vi "Lab Panel V4.91.vi"() -> ()   [LabVIEW 2013] (continued)
                n1771 = property on="SET LAB03-2" class="Clust (strict)"("DisabledEnum"=w3330) -> ()  [unwired: 2 in, 2 out]
                n1772 = property on="SET LAB04-1" class="Clust (strict)"("DisabledEnum"=w3329) -> ()  [unwired: 2 in, 2 out]
                n1773 = property on="SET LAB04-2" class="Clust (strict)"("DisabledEnum"=w3328) -> ()  [unwired: 2 in, 2 out]
                n1774 = property on="O/I  LAB05-2" class="Bool (strict)"("DisabledEnum"=w3326) -> ()  [unwired: 2 in, 2 out]
                n1775 = property on="O/I  LAB05-1" class="Bool (strict)"("DisabledEnum"=w3327) -> ()  [unwired: 2 in, 2 out]
                n1776 = property on="O/I  LAB04-1" class="Bool (strict)"("DisabledEnum"=w3329) -> ()  [unwired: 2 in, 2 out]
                n1777 = property on="O/I  LAB04-2" class="Bool (strict)"("DisabledEnum"=w3328) -> ()  [unwired: 2 in, 2 out]
                n1778 = property on="O/I  LAB03-2" class="Bool (strict)"("DisabledEnum"=w3330) -> ()  [unwired: 2 in, 2 out]
                n1779 = Not(x=w3335) -> (.not. x?=w3336:bool)
                n1780 = Not(x=w3334) -> (.not. x?=w3337:bool)
                n1781 = Not(x=w3333) -> (.not. x?=w3338:bool)
                n1782 = property on="RESULT LAB05-2" class="Bool (strict)"("Visible"=w3336) -> ()  [unwired: 2 in, 2 out]
                n1783 = property on="RESULT LAB05-1" class="Bool (strict)"("Visible"=w3337) -> ()  [unwired: 2 in, 2 out]
                n1784 = Not(x=w3332) -> (.not. x?=w3339:bool)
                n1785 = property on="RESULT LAB04-2" class="Bool (strict)"("Visible"=w3338) -> ()  [unwired: 2 in, 2 out]
                n1786 = Not(x=w3331) -> (.not. x?=w3340:bool)
                n1787 = property on="RESULT LAB04-1" class="Bool (strict)"("Visible"=w3339) -> ()  [unwired: 2 in, 2 out]
                n1788 = property on="RESULT LAB03-2" class="Bool (strict)"("Visible"=w3340) -> ()  [unwired: 2 in, 2 out]
              }
              frame #2 {
                # "disable calibrate if any test running"
                n1789 = Or(x=w3363, y=w3362) -> (x .or. y?=w3356:bool)
                n1790 = Or(x=w3365, y=w3364) -> (x .or. y?=w3358:bool)
                n1791 = Or(x=w3369, y=w3368) -> (x .or. y?=w3360:bool)
                n1792 = Or(x=w3367, y=w3366) -> (x .or. y?=w3359:bool)
                n1793 = Or(x=w3371, y=w3370) -> (x .or. y?=w3361:bool)
                n1794 = Or(x=w3359, y=w3358) -> (x .or. y?=w3357:bool)
                n1795 = Or(x=w3361, y=w3360) -> (x .or. y?=w3355:bool)
                n1796 = Or(x=w3357, y=w3356) -> (x .or. y?=w3354:bool)
                n1797 = Or(x=w3355, y=w3354) -> (x .or. y?=w3353:bool)
                n1798 = case shown="False" w3353 {
                  tunnel: [0 2] -> w3352
                  frame False {
                  }
                  frame True {
                  }
                }
                n1799 = property on="JIG TEST" class="Clust (strict)"("DisabledEnum"=w3352) -> ()  [unwired: 2 in, 2 out]
                n1800 = property on="Network Directory" class="Path"("DisabledEnum"=w3352) -> ()  [unwired: 2 in, 2 out]
                n1801 = property on="MAIL SETTINGS" class="Clust (strict)"("DisabledEnum"=w3352) -> ()  [unwired: 2 in, 2 out]
                n1802 = property on="SET (cal)" class="Bool (strict)"("DisabledEnum"=w3352) -> ()  [unwired: 2 in, 2 out]
                n1803 = property on="ADMIN" class="Bool (strict)"("DisabledEnum"=0) -> ()  [unwired: 2 in, 2 out]
              }
            }
          }
          frame #8 {
            # "drive jigs"
            n1804 = stacked-sequence {
              frame #0 {
                # "jig on"
                n1805 = local read "jig cycle"() -> (w3379:dbl)
                n1806 = property on="JIG TEST" class="Clust (strict)"() -> ("DisabledEnum"=w3376:T16)  [unwired: 2 in, 2 out]
                n1807 = Equal?(x=w3376, y=2) -> (x = y?=w3375:bool)
                n1808 = Equal?(x=w3379, y=0) -> (x = y?=w3377:bool)
                n1809 = And(x=w3377, y=w3375) -> (x .and. y?=w3374:bool)
                n1810 = case shown="True" w3374 {
                  frame False {
                  }
                  frame True {
                    n1811 = local read "run lab01-1"() -> (w3390:bool)
                    n1812 = local read "run lab01-2"() -> (w3389:bool)
                    n1813 = local read "run lab02-1"() -> (w3388:bool)
                    n1814 = local read "run lab02-2"() -> (w3387:bool)
                    n1815 = local read "run lab03-1"() -> (w3386:bool)
                    n1816 = local read "run lab03-2"() -> (w3385:bool)
                    n1817 = local read "run lab04-1"() -> (w3384:bool)
                    n1818 = local read "run lab04-2"() -> (w3383:bool)
                    n1819 = local read "run lab05-1"() -> (w3382:bool)
                    n1820 = local read "run lab05-2"() -> (w3381:bool)
                    n1821 = local write "JIG LAB03-2"(w3385) -> ()
                    n1822 = local write "JIG LAB01-1"(w3390) -> ()
                    n1823 = local write "JIG LAB01-2"(w3389) -> ()
                    n1824 = local write "JIG LAB02-1"(w3388) -> ()
                    n1825 = local write "JIG LAB02-2"(w3387) -> ()
                    n1826 = local write "JIG LAB03-1"(w3386) -> ()
                    n1827 = local write "JIG LAB04-1"(w3384) -> ()
                    n1828 = local write "JIG LAB04-2"(w3383) -> ()
                    n1829 = local write "JIG LAB05-1"(w3382) -> ()
                    n1830 = local write "JIG LAB05-2"(w3381) -> ()
                  }
                }
              }
              frame #1 {
                # "jig off"
                n1831 = local read "jig cycle"() -> (w3397:dbl)
                n1832 = local read "on loops"() -> (w3396:dbl)
                n1833 = property on="JIG TEST" class="Clust (strict)"() -> ("DisabledEnum"=w3395:T16)  [unwired: 2 in, 2 out]
                n1834 = Equal?(x=w3395, y=2) -> (x = y?=w3393:bool)
                n1835 = Equal?(x=w3397, y=w3396) -> (x = y?=w3392:bool)
                n1836 = And(x=w3392, y=w3393) -> (x .and. y?=w3391:bool)
                n1837 = case shown="True" w3391 {
                  frame False {
                  }
                  frame True {
                    w3448 = FALSE
                    w3449 = TRUE
                    w3447 = 2
                    n1838 = local read "SELECT LAB05-2"() -> (w3438:T3)
                    n1839 = local read "SELECT LAB04-2"() -> (w3440:T3)
                    n1840 = local read "SELECT LAB04-1"() -> (w3441:T3)
                    n1841 = local read "SELECT LAB05-1"() -> (w3439:T3)
                    n1842 = local read "SELECT LAB03-2"() -> (w3442:T3)
                    n1843 = local read "SELECT LAB02-1"() -> (w3445:T3)
                    n1844 = local read "SELECT LAB03-1"() -> (w3443:T3)
                    n1845 = local read "SELECT LAB02-2"() -> (w3444:T3)
                    n1846 = local read "SELECT LAB01-2"() -> (w3446:T3)
                    n1847 = local read "run lab05-1"() -> (w3408:bool)
                    n1848 = local read "run lab05-2"() -> (w3407:bool)
                    n1849 = local read "SELECT LAB01-1"() -> (w3450:T3)
                    n1850 = local read "run lab04-2"() -> (w3409:bool)
                    n1851 = local read "run lab04-1"() -> (w3410:bool)
                    n1852 = local read "run lab01-1"() -> (w3426:bool)
                    n1853 = local read "run lab01-2"() -> (w3415:bool)
                    n1854 = local read "run lab03-2"() -> (w3411:bool)
                    n1855 = local read "run lab03-1"() -> (w3412:bool)
                    n1856 = local read "run lab02-1"() -> (w3414:bool)
                    n1857 = local read "run lab02-2"() -> (w3413:bool)
                    n1858 = Equal?(x=w3447, y=w3443) -> (x = y?=w3421:bool)
                    n1859 = Equal?(x=w3447, y=w3442) -> (x = y?=w3420:bool)
                    n1860 = Equal?(x=w3447, y=w3441) -> (x = y?=w3419:bool)
                    n1861 = Equal?(x=w3447, y=w3440) -> (x = y?=w3418:bool)
                    n1862 = Equal?(x=w3447, y=w3439) -> (x = y?=w3417:bool)
                    n1863 = Equal?(x=w3447, y=w3438) -> (x = y?=w3416:bool)
                    n1864 = Equal?(x=w3447, y=w3450) -> (x = y?=w3427:bool)
                    n1865 = Equal?(x=w3447, y=w3445) -> (x = y?=w3423:bool)
                    n1866 = Equal?(x=w3447, y=w3444) -> (x = y?=w3422:bool)
                    n1867 = Equal?(x=w3447, y=w3446) -> (x = y?=w3424:bool)
                    n1868 = And(x=w3418, y=w3409) -> (x .and. y?=w3400:bool)
                    n1869 = And(x=w3421, y=w3412) -> (x .and. y?=w3403:bool)
                    n1870 = And(x=w3419, y=w3410) -> (x .and. y?=w3401:bool)
                    n1871 = And(x=w3416, y=w3407) -> (x .and. y?=w3398:bool)
                    n1872 = And(x=w3422, y=w3413) -> (x .and. y?=w3404:bool)
                    n1873 = And(x=w3420, y=w3411) -> (x .and. y?=w3402:bool)
                    n1874 = And(x=w3417, y=w3408) -> (x .and. y?=w3399:bool)
                    n1875 = And(x=w3424, y=w3415) -> (x .and. y?=w3406:bool)
                    n1876 = And(x=w3427, y=w3426) -> (x .and. y?=w3425:bool)
                    n1877 = And(x=w3423, y=w3414) -> (x .and. y?=w3405:bool)
                    n1878 = Select(t=w3449, s=w3425, f=w3448) -> (s? t:f=w3428:bool)
                    n1879 = Select(t=w3449, s=w3406, f=w3448) -> (s? t:f=w3429:bool)
                    n1880 = Select(t=w3449, s=w3405, f=w3448) -> (s? t:f=w3430:bool)
                    n1881 = Select(t=w3449, s=w3404, f=w3448) -> (s? t:f=w3431:bool)
                    n1882 = Select(t=w3449, s=w3403, f=w3448) -> (s? t:f=w3432:bool)
                    n1883 = Select(t=w3449, s=w3402, f=w3448) -> (s? t:f=w3433:bool)
                    n1884 = Select(t=w3449, s=w3401, f=w3448) -> (s? t:f=w3434:bool)
                    n1885 = Select(t=w3449, s=w3400, f=w3448) -> (s? t:f=w3435:bool)
                    n1886 = Select(t=w3449, s=w3399, f=w3448) -> (s? t:f=w3436:bool)
                    n1887 = Select(t=w3449, s=w3398, f=w3448) -> (s? t:f=w3437:bool)
                    n1888 = local write "JIG LAB03-2"(w3433) -> ()
                    n1889 = local write "JIG LAB02-1"(w3430) -> ()
                    n1890 = local write "JIG LAB02-2"(w3431) -> ()
                    n1891 = local write "JIG LAB01-2"(w3429) -> ()
                    n1892 = local write "JIG LAB03-1"(w3432) -> ()
                    n1893 = local write "JIG LAB01-1"(w3428) -> ()
                    n1894 = local write "JIG LAB05-2"(w3437) -> ()
                    n1895 = local write "JIG LAB04-1"(w3434) -> ()
                    n1896 = local write "JIG LAB05-1"(w3436) -> ()
                    n1897 = local write "JIG LAB04-2"(w3435) -> ()
                  }
                }
              }
            }
          }
          frame #9 {
            # "enable  jig test output if no test busy"
            n1898 = property on="JIG TEST" class="Clust (strict)"() -> ("DisabledEnum"=w3453:T16)  [unwired: 2 in, 2 out]
            n1899 = Equal?(x=w3453, y=0) -> (x = y?=w3451:bool)
            n1900 = case shown="True" w3451 {
              frame False {
              }
              frame True {
                n1901 = local read "JIG TEST"() -> (w3464:T10)
                n1902 = Unbundle(w3464) -> ("LAB01-1"=w3463:bool, "LAB01-2"=w3462:bool, "LAB02-1"=w3461:bool, "LAB02-2"=w3460:bool, "LAB03-1"=w3459:bool, "LAB03-2"=w3458:bool, "LAB04-1"=w3457:bool, "LAB04-2"=w3456:bool, "LAB05-1"=w3455:bool, "LAB05-2"=w3454:bool)
                n1903 = local write "JIG LAB05-1"(w3455) -> ()
                n1904 = local write "JIG LAB05-2"(w3454) -> ()
                n1905 = local write "JIG LAB04-1"(w3457) -> ()
                n1906 = local write "JIG LAB04-2"(w3456) -> ()
                n1907 = local write "JIG LAB03-2"(w3458) -> ()
                n1908 = local write "JIG LAB01-1"(w3463) -> ()
                n1909 = local write "JIG LAB02-1"(w3461) -> ()
                n1910 = local write "JIG LAB03-1"(w3459) -> ()
                n1911 = local write "JIG LAB01-2"(w3462) -> ()
                n1912 = local write "JIG LAB02-2"(w3460) -> ()
              }
            }
          }
          frame #10 {
            # "drive digital output"
            n1913 = local read "O/I  LAB05-2"() -> (w3471:bool)
            n1914 = local read "O/I  LAB05-1"() -> (w3473:bool)
            n1915 = local read "JIG LAB05-2"() -> (w3470:bool)
            n1916 = local read "O/I  LAB04-2"() -> (w3475:bool)
            n1917 = local read "JIG LAB05-1"() -> (w3472:bool)
            n1918 = local read "JIG LAB04-2"() -> (w3474:bool)
            n1919 = local read "O/I  LAB03-1"() -> (w3480:bool)
            n1920 = local read "O/I  LAB04-1"() -> (w3476:bool)
            n1921 = local read "O/I  LAB02-1"() -> (w3484:bool)
            n1922 = local read "O/I  LAB02-2"() -> (w3482:bool)
            n1923 = local read "O/I  LAB03-2"() -> (w3478:bool)
            n1924 = local read "JIG LAB04-1"() -> (w3469:bool)
            n1925 = local read "JIG LAB03-2"() -> (w3477:bool)
            n1926 = local read "O/I  LAB01-2"() -> (w3486:bool)
            n1927 = local read "JIG LAB02-1"() -> (w3483:bool)
            n1928 = local read "JIG LAB02-2"() -> (w3481:bool)
            n1929 = local read "JIG LAB03-1"() -> (w3479:bool)
            n1930 = local read "O/I  LAB01-1"() -> (w3488:bool)
            n1931 = local read "JIG LAB01-2"() -> (w3485:bool)
            n1932 = local read "JIG LAB01-1"() -> (w3487:bool)
            n1933 = Build Array(w3475, w3474, w3473, w3472, w3471, w3470) -> (w3466:bool[])
            n1934 = Build Array(w3481, w3480, w3479, w3478, w3477, w3476, w3469) -> (w3467:bool[])
            n1935 = Build Array(w3488, w3487, w3486, w3485, w3484, w3483, w3482) -> (w3468:bool[])
            n1936 = local read "simulate"() -> (w3465:bool)
            n1937 = case shown="False" w3465 {
              tunnel: w3468 -> [w3491 _]
              tunnel: w3467 -> [w3490 _]
              tunnel: w3466 -> [w3489 _]
              frame False {
                n1938 = call "sub vi - Drive Relays All v6.vi"("Array #2"=w3489, "Array #1"=w3490, "Array #0"=w3491) -> ()  [unwired: 8 in, 1 out]
              }
              frame True {
              }
            }
          }
          frame #11 {
            # "get analog values"
            n1939 = local read "on loops"() -> (w3498:dbl)
            n1940 = local read "jig cycle"() -> (w3495:dbl)
            n1941 = Add(x=w3498, y=1) -> (x+y=w3496:dbl)
            n1942 = Equal?(x=w3495, y=1) -> (x = y?=w3492:bool)
            n1943 = Equal?(x=w3495, y=w3496) -> (x = y?=w3494:bool)
            n1944 = Or(x=w3492, y=w3494) -> (x .or. y?=w3493:bool)
            n1945 = global write "Global display 3.vi" "cycle O/F"(w3492) -> ()
            n1946 = case shown="True" w3493 {
              tunnel: w3492 -> [_ w3501]
              frame False {
              }
              frame True {
                n1947 = local read "simulate"() -> (w3504:bool)
                n1948 = case shown="False" w3504 {
                  tunnel: [errorcluster[] [] ("array ERROR") errorcluster[] [] ("array ERROR")] -> w3512
                  tunnel: [w3521 0.3 ("Analog loop time")] -> w3511
                  tunnel: [w3520 dynamicdata[] [] ("array GRAPH")] -> w3510
                  tunnel: [w3519 w3525] -> w3509
                  tunnel: [w3518 w3525] -> w3508
                  tunnel: [w3517 w3525] -> w3507
                  tunnel: [w3516 w3525] -> w3506
                  tunnel: [w3515 w3525] -> w3505
                  tunnel: w3501 -> [_ w3529]
                  tunnel: [w3514 2.92] -> w3500
                  frame False {
                    n1949 = call "sub vi - Read Analog All v9.11.vi"() -> ("Analog loop time"=w3521:dbl, "array GRAPH"=w3520:dynamicdata[], "LAB01"=w3519:T26, "LAB02"=w3518:T27, "LAB03"=w3517:T28, "LAB04"=w3516:T29, "deg C"=w3514:dbl, "LAB05"=w3515:T30)  [unwired: 7 in, 1 out]
                  }
                  frame True {
                    n1950 = local read "ON amps"() -> (w3522:dbl)
                    n1951 = local read "OFF amps"() -> (w3523:dbl)
                    n1952 = local read "VOLTS"() -> (w3527:dbl)
                    n1953 = local read "PF"() -> (w3526:dbl)
                    n1954 = Select(t=w3522, s=w3529, f=w3523) -> (s? t:f=w3528:dbl)
                    n1955 = Bundle("OFF amps"=w3528, "VOLTS"=w3527, "PF"=w3526, "OFF amps"=w3528, "VOLTS"=w3527, "PF"=w3526) -> (w3525:T31)  [unwired: 1 in]
                  }
                }
                n1956 = local read "simulate"() -> (w3503:bool)
                n1957 = stacked-sequence {
                  tunnel: w3512 -> [w3537 _ _ _ _ _ _]
                  tunnel: w3511 -> [w3536 _ _ _ _ _ _]
                  tunnel: w3510 -> [w3533 _ _ _ _ _ _]
                  tunnel: w3509 -> [_ w3584 _ _ _ _ _]
                  tunnel: w3508 -> [_ _ w3591 _ _ _ _]
                  tunnel: w3507 -> [_ _ _ w3620 _ _ _]
                  tunnel: w3506 -> [_ _ _ _ w3647 _ _]
                  tunnel: w3505 -> [_ _ _ _ _ w3676 _]
                  tunnel: w3503 -> [_ w3562 w3590 w3618 w3646 w3674 w3700]
                  tunnel: T14 {"1  (A) cal"=1.0, "1 (V) cal"=1.0, "1 (PF) cal"=1.0, "1 (TL) cal"=1.0, "1 (TN) cal"=1.0, "2 (A) cal"=1.0, "2 (V) cal"=1.0, "2 (PF) cal"=1.0, "2 (TL) cal"=1.0, "2 (TN) cal"=1.0} ("CAL LAB01") -> [_ w3561 w3589 w3617 w3645 w3673 _]
                  tunnel: w3500 -> [_ _ _ _ _ _ w3699]
                  frame #0 {
                    n1958 = local write "AI"(TRUE) -> ()
                    n1959 = global write "Global 1.vi" "RATE(Hz)"("RATE (Hz)") -> ()
                    n1960 = global write "Global 1.vi" "SAMPLES"("SAMPLES") -> ()
                    n1961 = Index Array(array=w3533, index=6) -> (element=→"LAB04-1 (GRAPH)":dynamicdata)
                    n1962 = Index Array(array=w3533, index=7) -> (element=→"LAB04-2 (GRAPH)":dynamicdata)
                    n1963 = Index Array(array=w3533, index=9) -> (element=→"LAB05-2 (GRAPH)":dynamicdata)
                    n1964 = Index Array(array=w3533, index=8) -> (element=→"LAB05-1 (GRAPH)":dynamicdata)
                    n1965 = Index Array(array=w3533, index=5) -> (element=→"LAB03-2 (GRAPH)":dynamicdata)
                    n1966 = Index Array(array=w3533, index=0) -> (element=→"LAB01-1 (GRAPH)":dynamicdata)
                    n1967 = Index Array(array=w3533, index=1) -> (element=→"LAB01-2 (GRAPH)":dynamicdata)
                    n1968 = Index Array(array=w3533, index=2) -> (element=→"LAB02-1 (GRAPH)":dynamicdata)
                    n1969 = Index Array(array=w3533, index=3) -> (element=→"LAB02-2 (GRAPH)":dynamicdata)
                    n1970 = Index Array(array=w3533, index=4) -> (element=→"LAB03-1 (GRAPH)":dynamicdata)
                    "AI loop time" <- w3536
                    "Analog Error Array" <- w3537
                  }
                  frame #1 {
                    n1971 = case shown="False" w3562 {
                      tunnel: [w3585 w3586] -> w3583
                      tunnel: w3561 -> [_ w3586]
                      frame False {
                        n1972 = local read "CAL LAB01"() -> (w3585:T14)
                      }
                      frame True {
                      }
                    }
                    n1973 = Unbundle By Name(w3584) -> ("OFF amps"=w3582:dbl, "VOLTS"=w3581:dbl, "PF"=w3580:dbl, "OFF amps"=w3579:dbl, "VOLTS"=w3578:dbl, "PF"=w3577:dbl)
                    n1974 = Unbundle By Name(w3583) -> ("1  (A) cal"=w3576:dbl, "1 (V) cal"=w3575:dbl, "1 (PF) cal"=w3574:dbl, "2 (A) cal"=w3573:dbl, "2 (V) cal"=w3572:dbl, "2 (PF) cal"=w3571:dbl)  [unwired: 4 out]
                    n1975 = Multiply(x=w3582, y=w3576) -> (x*y=w3569:dbl)
                    n1976 = Multiply(x=w3581, y=w3575) -> (x*y=w3568:dbl)
                    n1977 = Multiply(x=w3580, y=w3574) -> (x*y=w3567:dbl)
                    n1978 = Multiply(x=w3579, y=w3573) -> (x*y=w3565:dbl)
                    n1979 = Multiply(x=w3578, y=w3572) -> (x*y=w3564:dbl)
                    n1980 = Multiply(x=w3577, y=w3571) -> (x*y=w3563:dbl)
                    n1981 = local read "SIG LAB01-1"() -> (w3570:T2)
                    n1982 = local read "SIG LAB01-2"() -> (w3566:T2)
                    n1983 = Bundle By Name(cluster=w3570, "AMPS"=w3569, "VOLTS"=w3568, "PF"=w3567) -> (w3560:T2)
                    n1984 = Bundle By Name(cluster=w3566, "AMPS"=w3565, "VOLTS"=w3564, "PF"=w3563) -> (w3559:T2)
                    n1985 = global write "Global display 1.vi" "SIG LAB01-2"(w3559) -> ()
                    n1986 = global write "Global display 1.vi" "SIG LAB01-1"(w3560) -> ()
                    n1987 = local write "SIG LAB01-2"(w3559) -> ()
                    n1988 = local write "SIG LAB01-1"(w3560) -> ()
                  }
                  frame #2 {
                    n1989 = Unbundle By Name(w3591) -> ("OFF amps"=w3611:dbl, "VOLTS"=w3610:dbl, "PF"=w3609:dbl, "OFF amps"=w3608:dbl, "VOLTS"=w3607:dbl, "PF"=w3606:dbl)
                    n1990 = case shown="True" w3590 {
                      tunnel: [w3613 w3614] -> w3612
                      tunnel: w3589 -> [_ w3614]
                      frame False {
                        n1991 = local read "CAL LAB02"() -> (w3613:T15)
                      }
                      frame True {
                      }
                    }
                    n1992 = Unbundle By Name(w3612) -> ("1  (A) cal"=w3605:dbl, "1 (V) cal"=w3604:dbl, "1 (PF) cal"=w3603:dbl, "2 (A) cal"=w3602:dbl, "2 (V) cal"=w3601:dbl, "2 (PF) cal"=w3600:dbl)  [unwired: 4 out]
                    n1993 = Multiply(x=w3611, y=w3605) -> (x*y=w3598:dbl)
                    n1994 = Multiply(x=w3610, y=w3604) -> (x*y=w3597:dbl)
                    n1995 = Multiply(x=w3609, y=w3603) -> (x*y=w3596:dbl)
                    n1996 = Multiply(x=w3608, y=w3602) -> (x*y=w3594:dbl)
                    n1997 = Multiply(x=w3607, y=w3601) -> (x*y=w3593:dbl)
                    n1998 = Multiply(x=w3606, y=w3600) -> (x*y=w3592:dbl)
                    n1999 = local read "SIG LAB02-1"() -> (w3599:T2)
                    n2000 = local read "SIG LAB02-2"() -> (w3595:T2)
                    n2001 = Bundle By Name(cluster=w3599, "AMPS"=w3598, "VOLTS"=w3597, "PF"=w3596) -> (w3588:T2)
                    n2002 = Bundle By Name(cluster=w3595, "AMPS"=w3594, "VOLTS"=w3593, "PF"=w3592) -> (w3587:T2)
                    n2003 = global write "Global display 1.vi" "SIG LAB02-1"(w3588) -> ()
                    n2004 = local write "SIG LAB02-2"(w3587) -> ()
                    n2005 = global write "Global display 1.vi" "SIG LAB02-2"(w3587) -> ()
                    n2006 = local write "SIG LAB02-1"(w3588) -> ()
                  }
                  frame #3 {
                    n2007 = Unbundle By Name(w3620) -> ("OFF amps"=w3639:dbl, "VOLTS"=w3638:dbl, "PF"=w3637:dbl, "OFF amps"=w3636:dbl, "VOLTS"=w3635:dbl, "PF"=w3634:dbl)
                    n2008 = case shown="True" w3618 {
                      tunnel: [w3641 w3642] -> w3640
                      tunnel: w3617 -> [_ w3642]
                      frame False {
                        n2009 = local read "CAL LAB03"() -> (w3641:T14)
                      }
                      frame True {
                      }
                    }
                    n2010 = Unbundle By Name(w3640) -> ("1  (A) cal"=w3633:dbl, "1 (V) cal"=w3632:dbl, "1 (PF) cal"=w3631:dbl, "2 (A) cal"=w3630:dbl, "2 (V) cal"=w3629:dbl, "2 (PF) cal"=w3628:dbl)  [unwired: 4 out]
                    n2011 = Multiply(x=w3639, y=w3633) -> (x*y=w3626:dbl)
                    n2012 = Multiply(x=w3638, y=w3632) -> (x*y=w3619:dbl)
                    n2013 = Multiply(x=w3637, y=w3631) -> (x*y=w3625:dbl)
                    n2014 = Multiply(x=w3636, y=w3630) -> (x*y=w3623:dbl)
                    n2015 = Multiply(x=w3635, y=w3629) -> (x*y=w3622:dbl)
                    n2016 = Multiply(x=w3634, y=w3628) -> (x*y=w3621:dbl)
                    n2017 = local read "SIG LAB03-1"() -> (w3627:T2)
                    n2018 = local read "SIG LAB03-2"() -> (w3624:T2)
                    n2019 = Bundle By Name(cluster=w3627, "AMPS"=w3626, "VOLTS"=w3619, "PF"=w3625) -> (w3616:T2)
                    n2020 = Bundle By Name(cluster=w3624, "AMPS"=w3623, "VOLTS"=w3622, "PF"=w3621) -> (w3615:T2)
                    n2021 = global write "Global display 1.vi" "SIG LAB03-1"(w3616) -> ()
                    n2022 = global write "Global display 1.vi" "SIG LAB03-2"(w3615) -> ()
                    n2023 = local write "SIG LAB03-2"(w3615) -> ()
                    n2024 = local write "SIG LAB03-1"(w3616) -> ()
                  }
                  frame #4 {
                    n2025 = Unbundle By Name(w3647) -> ("OFF amps"=w3667:dbl, "VOLTS"=w3666:dbl, "PF"=w3665:dbl, "OFF amps"=w3664:dbl, "VOLTS"=w3663:dbl, "PF"=w3662:dbl)
                    n2026 = case shown="False" w3646 {
                      tunnel: [w3669 w3670] -> w3668
                      tunnel: w3645 -> [_ w3670]
                      frame False {
                        n2027 = local read "CAL LAB04"() -> (w3669:T14)
                      }
                      frame True {
                      }
                    }
                    n2028 = Unbundle By Name(w3668) -> ("1  (A) cal"=w3661:dbl, "1 (V) cal"=w3660:dbl, "1 (PF) cal"=w3659:dbl, "2 (A) cal"=w3658:dbl, "2 (V) cal"=w3657:dbl, "2 (PF) cal"=w3656:dbl)  [unwired: 4 out]
                    n2029 = Multiply(x=w3667, y=w3661) -> (x*y=w3654:dbl)
                    n2030 = Multiply(x=w3666, y=w3660) -> (x*y=w3653:dbl)
                    n2031 = Multiply(x=w3665, y=w3659) -> (x*y=w3652:dbl)
                    n2032 = Multiply(x=w3664, y=w3658) -> (x*y=w3650:dbl)
                    n2033 = Multiply(x=w3663, y=w3657) -> (x*y=w3649:dbl)
                    n2034 = Multiply(x=w3662, y=w3656) -> (x*y=w3648:dbl)
                    n2035 = local read "SIG LAB04-1"() -> (w3655:T2)
                    n2036 = local read "SIG LAB04-2"() -> (w3651:T2)
                    n2037 = Bundle By Name(cluster=w3655, "AMPS"=w3654, "VOLTS"=w3653, "PF"=w3652) -> (w3644:T2)
                    n2038 = Bundle By Name(cluster=w3651, "AMPS"=w3650, "VOLTS"=w3649, "PF"=w3648) -> (w3643:T2)
                    n2039 = global write "Global display 1.vi" "SIG LAB04-2"(w3643) -> ()
                    n2040 = global write "Global display 1.vi" "SIG LAB04-1"(w3644) -> ()
                    n2041 = local write "SIG LAB04-2"(w3643) -> ()
                    n2042 = local write "SIG LAB04-1"(w3644) -> ()
                  }
                  frame #5 {
                    n2043 = Unbundle By Name(w3676) -> ("OFF amps"=w3695:dbl, "VOLTS"=w3675:dbl, "PF"=w3694:dbl, "OFF amps"=w3693:dbl, "VOLTS"=w3692:dbl, "PF"=w3691:dbl)
                    n2044 = case shown="False" w3674 {
                      tunnel: [w3697 w3698] -> w3696
                      tunnel: w3673 -> [_ w3698]
                      frame False {
                        n2045 = local read "CAL LAB05"() -> (w3697:T14)
                      }
                      frame True {
                      }
                    }
                    n2046 = Unbundle By Name(w3696) -> ("1  (A) cal"=w3690:dbl, "1 (V) cal"=w3689:dbl, "1 (PF) cal"=w3688:dbl, "2 (A) cal"=w3687:dbl, "2 (V) cal"=w3686:dbl, "2 (PF) cal"=w3685:dbl)  [unwired: 4 out]
                    n2047 = Multiply(x=w3695, y=w3690) -> (x*y=w3683:dbl)
                    n2048 = Multiply(x=w3675, y=w3689) -> (x*y=w3682:dbl)
                    n2049 = Multiply(x=w3694, y=w3688) -> (x*y=w3681:dbl)
                    n2050 = Multiply(x=w3693, y=w3687) -> (x*y=w3679:dbl)
                    n2051 = Multiply(x=w3692, y=w3686) -> (x*y=w3678:dbl)
                    n2052 = Multiply(x=w3691, y=w3685) -> (x*y=w3677:dbl)
                    n2053 = local read "SIG LAB05-1"() -> (w3684:T2)
                    n2054 = local read "SIG LAB05-2"() -> (w3680:T2)
                    n2055 = Bundle By Name(cluster=w3684, "AMPS"=w3683, "VOLTS"=w3682, "PF"=w3681) -> (w3672:T2)
                    n2056 = Bundle By Name(cluster=w3680, "AMPS"=w3679, "VOLTS"=w3678, "PF"=w3677) -> (w3671:T2)
                    n2057 = global write "Global display 1.vi" "SIG LAB05-1"(w3672) -> ()
                    n2058 = global write "Global display 1.vi" "SIG LAB05-2"(w3671) -> ()
                    n2059 = local write "SIG LAB05-2"(w3671) -> ()
                    n2060 = local write "SIG LAB05-1"(w3672) -> ()
                  }
                  frame #6 {
                    # "update ambient referance temperature"
                    n2061 = case shown="False" w3700 {
                      tunnel: [w3703 100.0] -> w3702
                      frame False {
                        n2062 = local read "TEMP REF cal"() -> (w3703:dbl)
                      }
                      frame True {
                      }
                    }
                    n2063 = local read "Panel #"() -> (w3701:dbl)
                    n2064 = case shown="1" w3701 {
                      tunnel: w3702 -> [_ w3709]
                      tunnel: w3699 -> [_ w3708]
                      frame 0, Default {
                      }
                      frame 1 {
                        n2065 = Multiply(x=w3709, y=w3708) -> (x*y=w3707:dbl)
                        n2066 = Subtract(x=w3707, y=272) -> (x-y=w3705:dbl)
                        "Amb Ref" <- w3705
                        n2067 = local write "Ref deg C"(w3705) -> ()
                      }
                    }
                    "deg C (volts)" <- w3699
                  }
                }
              }
            }
          }
          frame #12 {
            # "save test data to file"
            n2068 = Get Date/Time In Seconds() -> (seconds since 1Jan1904=w3710:timestamp)
            "File Time Stamp" <- w3710
            n2069 = local read "on loops"() -> (w3729:dbl)
            n2070 = local read "jig cycle"() -> (w3726:dbl)
            n2071 = Format Date/Time String(time format string (%c)="%H:%M%:%S", seconds (now)=w3710) -> (date/time string=w3714:string)  [unwired: 1 in]
            n2072 = Add(x=w3729, y=2) -> (x+y=w3727:dbl)
            n2073 = Build Array(w3714) -> (w3713:string[])
            n2074 = Equal?(x=w3726, y=1) -> (x = y?=w3712:bool)
            n2075 = Equal?(x=w3726, y=w3727) -> (x = y?=w3711:bool)
            n2076 = stacked-sequence {
              tunnel: w3725 -> [w3735 _ _ _ _ _ _ _ _ _]
              tunnel: w3724 -> [_ w3811 _ _ _ _ _ _ _ _]
              tunnel: w3723 -> [_ _ w3891 _ _ _ _ _ _ _]
              tunnel: w3722 -> [_ _ _ w3971 _ _ _ _ _ _]
              tunnel: w3721 -> [_ _ _ _ w4051 _ _ _ _ _]
              tunnel: w3720 -> [_ _ _ _ _ w4131 _ _ _ _]
              tunnel: w3719 -> [_ _ _ _ _ _ w4211 _ _ _]
              tunnel: w3718 -> [_ _ _ _ _ _ _ w4291 _ _]
              tunnel: w3717 -> [_ _ _ _ _ _ _ _ w4371 _]
              tunnel: w3716 -> [_ _ _ _ _ _ _ _ _ w4451]
              tunnel: w3713 -> [w3734 w3815 w3895 w3975 w4055 w4135 w4215 w4295 w4375 w4455]
              tunnel: w3712 -> [w3733 w3814 w3894 w3974 w4054 w4134 w4214 w4294 w4374 w4454]
              tunnel: w3711 -> [w3732 w3813 w3893 w3973 w4053 w4133 w4213 w4293 w4373 w4453]
              tunnel: w3710 -> [w3731 w3812 w3892 w3972 w4052 w4132 w4212 w4292 w4372 w4452]
              frame #0 {
                n2077 = case shown="True" w3735 {
                  tunnel: w3734 -> [_ w3740]
                  tunnel: w3733 -> [_ w3739]
                  tunnel: w3732 -> [_ w3737]
                  tunnel: w3731 -> [_ w3736]
                  frame False {
                  }
                  frame True {
                    n2078 = local read "DISP LAB01-1"() -> (w3741:T4)
                    n2079 = local read "SIG LAB01-1"() -> (w3742:T2)
                    n2080 = local read "ON L01-1"() -> (w3738:cluster{"amps":dbl, "volts":dbl, "pf":dbl})
                    n2081 = Unbundle(w3742) -> ("AMPS"=w3748:dbl, "VOLTS"=w3746:dbl, "PF"=w3745:dbl, "Tmp Live"=w3744:dbl, "Tmp Neut"=w3747:dbl)
                    n2082 = Unbundle(w3741) -> ("CYCLE"=w3743:dbl)  [unwired: 2 out]
                    n2083 = stacked-sequence {
                      tunnel: w3748 -> [w3752 w3771]
                      tunnel: w3747 -> [_ w3770]
                      tunnel: w3746 -> [w3751 w3769]
                      tunnel: w3745 -> [w3750 w3768]
                      tunnel: w3744 -> [_ w3767]
                      tunnel: w3743 -> [_ w3766]
                      tunnel: w3740 -> [_ w3765]
                      tunnel: w3739 -> [w3753 _]
                      tunnel: w3738 -> [w3749 w3763]
                      tunnel: w3737 -> [_ w3764]
                      tunnel: w3736 -> [_ w3759]
                      frame #0 {
                        n2084 = case shown="True" w3753 {
                          tunnel: w3752 -> [_ w3758]
                          tunnel: w3751 -> [_ w3757]
                          tunnel: w3750 -> [_ w3756]
                          tunnel: w3749 -> [_ w3754]
                          frame False {
                          }
                          frame True {
                            n2085 = Bundle(cluster=w3754, "amps"=w3758, "volts"=w3757, "pf"=w3756) -> (w3755:cluster{"amps":dbl, "volts":dbl, "pf":dbl})
                            n2086 = local write "ON L01-1"(w3755) -> ()
                          }
                        }
                      }
                      frame #1 {
                        n2087 = Unbundle(w3763) -> ("amps"=w3762:dbl, "volts"=w3761:dbl, "pf"=w3760:dbl)
                        n2088 = case shown="True" w3764 {
                          tunnel: w3771 -> [_ w3772]
                          tunnel: w3770 -> [_ w3810]
                          tunnel: w3769 -> [_ _]
                          tunnel: w3768 -> [_ _]
                          tunnel: w3767 -> [_ w3809]
                          tunnel: w3766 -> [_ w3808]
                          tunnel: w3765 -> [_ w3776]
                          tunnel: w3762 -> [_ w3773]
                          tunnel: w3761 -> [_ w3805]
                          tunnel: w3760 -> [_ w3804]
                          tunnel: w3759 -> [_ w3774]
                          frame False {
                          }
                          frame True {
                            n2089 = local read "TDMS LAB01-1"() -> (w3807:refnum<k34>)
                            n2090 = Build Array(w3805) -> (w3801:dbl[])
                            n2091 = Build Array(w3804) -> (w3800:dbl[])
                            n2092 = Build Array(w3809) -> (w3799:dbl[])
                            n2093 = Build Array(w3810) -> (w3798:dbl[])
                            n2094 = Build Array(w3773) -> (w3803:dbl[])
                            n2095 = Build Array(w3772) -> (w3802:dbl[])
                            n2096 = Build Array(w3808) -> (w3797:dbl[])
                            n2097 = Build Array("AMPS ON", "AMPS OFF", "VOLTS", "PF", "TEMP Live", "TEMP Neut", "CYCLE") -> (w3781:string[])
                            n2098 = Bundle By Name("Y"=w3803, "t0"=w3774) -> (w3796:waveform(dbl))  [unwired: 1 in]
                            n2099 = Bundle By Name("Y"=w3802, "t0"=w3774) -> (w3795:waveform(dbl))  [unwired: 1 in]
                            n2100 = Bundle By Name("Y"=w3801, "t0"=w3774) -> (w3794:waveform(dbl))  [unwired: 1 in]
                            n2101 = Bundle By Name("Y"=w3800, "t0"=w3774) -> (w3793:waveform(dbl))  [unwired: 1 in]
                            n2102 = Bundle By Name("Y"=w3799, "t0"=w3774) -> (w3792:waveform(dbl))  [unwired: 1 in]
                            n2103 = Bundle By Name("Y"=w3798, "t0"=w3774) -> (w3791:waveform(dbl))  [unwired: 1 in]
                            n2104 = Bundle By Name("Y"=w3797, "t0"=w3774) -> (w3790:waveform(dbl))  [unwired: 1 in]
                            n2105 = Build Array(w3796, w3795, w3794, w3793, w3792, w3791, w3790) -> (w3789:waveform(dbl)[])
                            n2106 = TDMS Write(0:w3807, 5:"TEST VALUES", 7:w3781, 9:w3789) -> (4:w3780:refnum<k34>, 6:w3779:string, 15:w3778:errorcluster)  [unwired: 2 in, 1 out]
                            n2107 = TDMS Write(0:w3780, 5:w3779, 7:"TIME", 9:w3776, 11:w3778) -> (15:w3775:errorcluster)  [unwired: 1 in, 3 out]
                            n2108 = local write "data file error"(w3775) -> ()
                          }
                        }
                      }
                    }
                  }
                }
              }
              frame #1 {
                n2109 = case shown="True" w3811 {
                  tunnel: w3815 -> [_ w3820]
                  tunnel: w3814 -> [_ w3819]
                  tunnel: w3813 -> [_ w3817]
                  tunnel: w3812 -> [_ w3816]
                  frame False {
                  }
                  frame True {
                    n2110 = local read "DISP LAB01-2"() -> (w3821:T4)
                    n2111 = local read "SIG LAB01-2"() -> (w3822:T2)
                    n2112 = local read "ON L01-2"() -> (w3818:cluster{"amps":dbl, "volts":dbl, "pf":dbl})
                    n2113 = Unbundle(w3822) -> ("AMPS"=w3828:dbl, "VOLTS"=w3826:dbl, "PF"=w3825:dbl, "Tmp Live"=w3824:dbl, "Tmp Neut"=w3827:dbl)
                    n2114 = Unbundle(w3821) -> ("CYCLE"=w3823:dbl)  [unwired: 2 out]
                    n2115 = stacked-sequence {
                      tunnel: w3828 -> [w3832 w3851]
                      tunnel: w3827 -> [_ w3850]
                      tunnel: w3826 -> [w3831 w3849]
                      tunnel: w3825 -> [w3830 w3848]
                      tunnel: w3824 -> [_ w3847]
                      tunnel: w3823 -> [_ w3846]
                      tunnel: w3820 -> [_ w3845]
                      tunnel: w3819 -> [w3833 _]
                      tunnel: w3818 -> [w3829 w3843]
                      tunnel: w3817 -> [_ w3844]
                      tunnel: w3816 -> [_ w3839]
                      frame #0 {
                        n2116 = case shown="True" w3833 {
                          tunnel: w3832 -> [_ w3838]
                          tunnel: w3831 -> [_ w3837]
                          tunnel: w3830 -> [_ w3836]
                          tunnel: w3829 -> [_ w3834]
                          frame False {
                          }
                          frame True {
                            n2117 = Bundle(cluster=w3834, "amps"=w3838, "volts"=w3837, "pf"=w3836) -> (w3835:cluster{"amps":dbl, "volts":dbl, "pf":dbl})
                            n2118 = local write "ON L01-2"(w3835) -> ()
                          }
                        }
                      }
                      frame #1 {
                        n2119 = Unbundle(w3843) -> ("amps"=w3842:dbl, "volts"=w3841:dbl, "pf"=w3840:dbl)
                        n2120 = case shown="True" w3844 {
                          tunnel: w3851 -> [_ w3883]
                          tunnel: w3850 -> [_ w3890]
                          tunnel: w3849 -> [_ _]
                          tunnel: w3848 -> [_ _]
                          tunnel: w3847 -> [_ w3889]
                          tunnel: w3846 -> [_ w3888]
                          tunnel: w3845 -> [_ w3853]
                          tunnel: w3842 -> [_ w3885]
                          tunnel: w3841 -> [_ w3884]
                          tunnel: w3840 -> [_ w3882]
                          tunnel: w3839 -> [_ w3874]
                          frame False {
                          }
                          frame True {
                            n2121 = local read "TDMS LAB01-2"() -> (w3887:refnum<k34>)
                            n2122 = Build Array(w3884) -> (w3879:dbl[])
                            n2123 = Build Array(w3882) -> (w3878:dbl[])
                            n2124 = Build Array(w3889) -> (w3877:dbl[])
                            n2125 = Build Array(w3890) -> (w3876:dbl[])
                            n2126 = Build Array(w3885) -> (w3881:dbl[])
                            n2127 = Build Array(w3883) -> (w3880:dbl[])
                            n2128 = Build Array(w3888) -> (w3875:dbl[])
                            n2129 = Build Array("AMPS ON", "AMPS OFF", "VOLTS", "PF", "TEMP Live", "TEMP Neut", "CYCLE") -> (w3858:string[])
                            n2130 = Bundle By Name("Y"=w3881, "t0"=w3874) -> (w3873:waveform(dbl))  [unwired: 1 in]
                            n2131 = Bundle By Name("Y"=w3880, "t0"=w3874) -> (w3872:waveform(dbl))  [unwired: 1 in]
                            n2132 = Bundle By Name("Y"=w3879, "t0"=w3874) -> (w3871:waveform(dbl))  [unwired: 1 in]
                            n2133 = Bundle By Name("Y"=w3878, "t0"=w3874) -> (w3870:waveform(dbl))  [unwired: 1 in]
                            n2134 = Bundle By Name("Y"=w3877, "t0"=w3874) -> (w3869:waveform(dbl))  [unwired: 1 in]
                            n2135 = Bundle By Name("Y"=w3876, "t0"=w3874) -> (w3868:waveform(dbl))  [unwired: 1 in]
                            n2136 = Bundle By Name("Y"=w3875, "t0"=w3874) -> (w3867:waveform(dbl))  [unwired: 1 in]
                            n2137 = Build Array(w3873, w3872, w3871, w3870, w3869, w3868, w3867) -> (w3866:waveform(dbl)[])
                            n2138 = TDMS Write(0:w3887, 5:"TEST VALUES", 7:w3858, 9:w3866) -> (4:w3857:refnum<k34>, 6:w3856:string, 15:w3855:errorcluster)  [unwired: 2 in, 1 out]
                            n2139 = TDMS Write(0:w3857, 5:w3856, 7:"TIME", 9:w3853, 11:w3855) -> (15:w3852:errorcluster)  [unwired: 1 in, 3 out]
                            n2140 = local write "data file error"(w3852) -> ()
                          }
                        }
                      }
                    }
                  }
                }
              }
              frame #2 {
                n2141 = case shown="True" w3891 {
                  tunnel: w3895 -> [_ w3900]
                  tunnel: w3894 -> [_ w3899]
                  tunnel: w3893 -> [_ w3897]
                  tunnel: w3892 -> [_ w3896]
                  frame False {
                  }
                  frame True {
                    n2142 = local read "DISP LAB02-1"() -> (w3901:T4)
                    n2143 = local read "SIG LAB02-1"() -> (w3902:T2)
                    n2144 = local read "ON L02-1"() -> (w3898:cluster{"amps":dbl, "volts":dbl, "pf":dbl})
                    n2145 = Unbundle(w3902) -> ("AMPS"=w3908:dbl, "VOLTS"=w3906:dbl, "PF"=w3905:dbl, "Tmp Live"=w3904:dbl, "Tmp Neut"=w3907:dbl)
                    n2146 = Unbundle(w3901) -> ("CYCLE"=w3903:dbl)  [unwired: 2 out]
                    n2147 = stacked-sequence {
                      tunnel: w3908 -> [w3912 w3931]
                      tunnel: w3907 -> [_ w3930]
                      tunnel: w3906 -> [w3911 w3929]
                      tunnel: w3905 -> [w3910 w3928]
                      tunnel: w3904 -> [_ w3927]
                      tunnel: w3903 -> [_ w3926]
                      tunnel: w3900 -> [_ w3925]
                      tunnel: w3899 -> [w3913 _]
                      tunnel: w3898 -> [w3909 w3923]
                      tunnel: w3897 -> [_ w3924]
                      tunnel: w3896 -> [_ w3919]
                      frame #0 {
                        n2148 = case shown="True" w3913 {
                          tunnel: w3912 -> [_ w3918]
                          tunnel: w3911 -> [_ w3917]
                          tunnel: w3910 -> [_ w3916]
                          tunnel: w3909 -> [_ w3914]
                          frame False {
                          }
                          frame True {
                            n2149 = Bundle(cluster=w3914, "amps"=w3918, "volts"=w3917, "pf"=w3916) -> (w3915:cluster{"amps":dbl, "volts":dbl, "pf":dbl})
                            n2150 = local write "ON L02-1"(w3915) -> ()
                          }
                        }
                      }
                      frame #1 {
                        n2151 = Unbundle(w3923) -> ("amps"=w3922:dbl, "volts"=w3921:dbl, "pf"=w3920:dbl)
                        n2152 = case shown="True" w3924 {
                          tunnel: w3931 -> [_ w3963]
                          tunnel: w3930 -> [_ w3970]
                          tunnel: w3929 -> [_ _]
                          tunnel: w3928 -> [_ _]
                          tunnel: w3927 -> [_ w3969]
                          tunnel: w3926 -> [_ w3968]
                          tunnel: w3925 -> [_ w3933]
                          tunnel: w3922 -> [_ w3965]
                          tunnel: w3921 -> [_ w3964]
                          tunnel: w3920 -> [_ w3962]
                          tunnel: w3919 -> [_ w3954]
                          frame False {
                          }
                          frame True {
                            n2153 = local read "TDMS LAB02-1"() -> (w3967:refnum<k34>)
                            n2154 = Build Array(w3964) -> (w3959:dbl[])
                            n2155 = Build Array(w3962) -> (w3958:dbl[])
                            n2156 = Build Array(w3969) -> (w3957:dbl[])
                            n2157 = Build Array(w3970) -> (w3956:dbl[])
                            n2158 = Build Array(w3965) -> (w3961:dbl[])
                            n2159 = Build Array(w3963) -> (w3960:dbl[])
                            n2160 = Build Array(w3968) -> (w3955:dbl[])
                            n2161 = Build Array("AMPS ON", "AMPS OFF", "VOLTS", "PF", "TEMP Live", "TEMP Neut", "CYCLE") -> (w3938:string[])
                            n2162 = Bundle By Name("Y"=w3961, "t0"=w3954) -> (w3953:waveform(dbl))  [unwired: 1 in]
                            n2163 = Bundle By Name("Y"=w3960, "t0"=w3954) -> (w3952:waveform(dbl))  [unwired: 1 in]
                            n2164 = Bundle By Name("Y"=w3959, "t0"=w3954) -> (w3951:waveform(dbl))  [unwired: 1 in]
                            n2165 = Bundle By Name("Y"=w3958, "t0"=w3954) -> (w3950:waveform(dbl))  [unwired: 1 in]
                            n2166 = Bundle By Name("Y"=w3957, "t0"=w3954) -> (w3949:waveform(dbl))  [unwired: 1 in]
                            n2167 = Bundle By Name("Y"=w3956, "t0"=w3954) -> (w3948:waveform(dbl))  [unwired: 1 in]
                            n2168 = Bundle By Name("Y"=w3955, "t0"=w3954) -> (w3947:waveform(dbl))  [unwired: 1 in]
                            n2169 = Build Array(w3953, w3952, w3951, w3950, w3949, w3948, w3947) -> (w3946:waveform(dbl)[])
                            n2170 = TDMS Write(0:w3967, 5:"TEST VALUES", 7:w3938, 9:w3946) -> (4:w3937:refnum<k34>, 6:w3936:string, 15:w3935:errorcluster)  [unwired: 2 in, 1 out]
                            n2171 = TDMS Write(0:w3937, 5:w3936, 7:"TIME", 9:w3933, 11:w3935) -> (15:w3932:errorcluster)  [unwired: 1 in, 3 out]
                            n2172 = local write "data file error"(w3932) -> ()
                          }
                        }
                      }
                    }
                  }
                }
              }
              frame #3 {
                n2173 = case shown="True" w3971 {
                  tunnel: w3975 -> [_ w3980]
                  tunnel: w3974 -> [_ w3979]
                  tunnel: w3973 -> [_ w3977]
                  tunnel: w3972 -> [_ w3976]
                  frame False {
                  }
                  frame True {
                    n2174 = local read "DISP LAB02-2"() -> (w3981:T4)
                    n2175 = local read "SIG LAB02-2"() -> (w3982:T2)
                    n2176 = local read "ON L02-2"() -> (w3978:cluster{"amps":dbl, "volts":dbl, "pf":dbl})
                    n2177 = Unbundle(w3982) -> ("AMPS"=w3988:dbl, "VOLTS"=w3986:dbl, "PF"=w3985:dbl, "Tmp Live"=w3984:dbl, "Tmp Neut"=w3987:dbl)
                    n2178 = Unbundle(w3981) -> ("CYCLE"=w3983:dbl)  [unwired: 2 out]
                    n2179 = stacked-sequence {
                      tunnel: w3988 -> [w3992 w4011]
                      tunnel: w3987 -> [_ w4010]
                      tunnel: w3986 -> [w3991 w4009]
                      tunnel: w3985 -> [w3990 w4008]
                      tunnel: w3984 -> [_ w4007]
                      tunnel: w3983 -> [_ w4006]
                      tunnel: w3980 -> [_ w4005]
                      tunnel: w3979 -> [w3993 _]
                      tunnel: w3978 -> [w3989 w4003]
                      tunnel: w3977 -> [_ w4004]
                      tunnel: w3976 -> [_ w3999]
                      frame #0 {
                        n2180 = case shown="True" w3993 {
                          tunnel: w3992 -> [_ w3998]
                          tunnel: w3991 -> [_ w3997]
                          tunnel: w3990 -> [_ w3996]
                          tunnel: w3989 -> [_ w3994]
                          frame False {
                          }
                          frame True {
                            n2181 = Bundle(cluster=w3994, "amps"=w3998, "volts"=w3997, "pf"=w3996) -> (w3995:cluster{"amps":dbl, "volts":dbl, "pf":dbl})
                            n2182 = local write "ON L02-2"(w3995) -> ()
                          }
                        }
                      }
                      frame #1 {
                        n2183 = Unbundle(w4003) -> ("amps"=w4002:dbl, "volts"=w4001:dbl, "pf"=w4000:dbl)
                        n2184 = case shown="True" w4004 {
                          tunnel: w4011 -> [_ w4043]
                          tunnel: w4010 -> [_ w4050]
                          tunnel: w4009 -> [_ _]
